vi "Temp_Calc.vi"(0 "aDATA":u8[](array[numeric])) -> (2 "Temp CH 1-4":dbl format="%#_3f", 3 "Temp CH 5-8":dbl, 4 "CPU Temp":dbl)   [LabVIEW 2010]
uses:
  <vilib>/Analysis/NI_AALPro.lvlib
panel:
  out "RT (Ohms) 2":dbl
  out "RT (Ohms)":dbl
  out "RT":dbl[](array[numeric]) format="%0.2f"
  out "Temp":dbl[](array[numeric]) format="%0.2f"
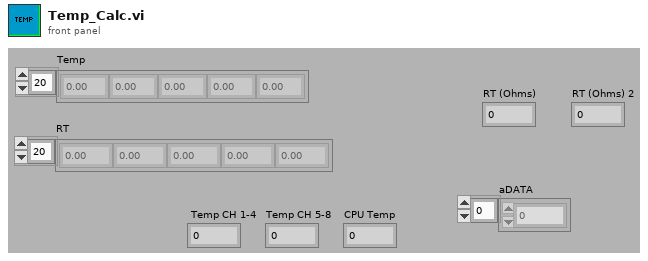
[diagram p1: front panel]
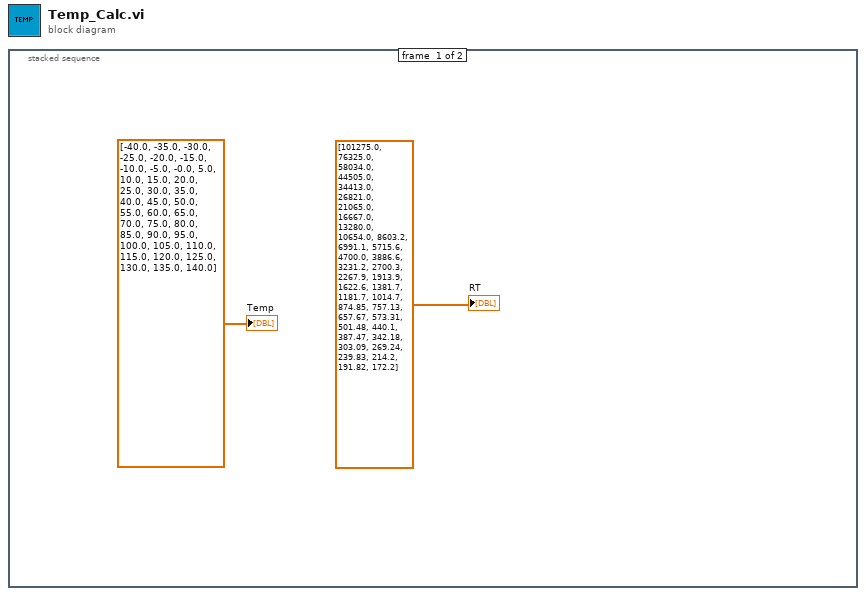
[diagram p0: block diagram]
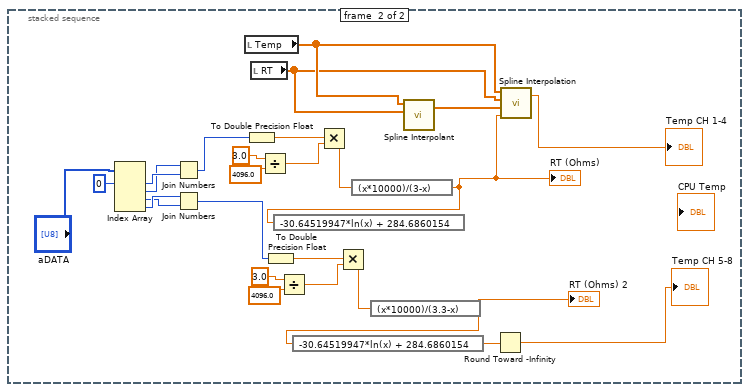
[diagram p2: hidden frame]
diagram:
  n1 = stacked-sequence {
    frame #0 {
      "Temp" <- dbl[] [-40.0, -35.0, -30.0, -25.0, -20.0, -15.0, -10.0, -5.0, -0.0, 5.0, 10.0, 15.0, 20.0, 25.0, 30.0, 35.0, 40.0, 45.0, 50.0, 55.0, 60.0, 65.0, 70.0, 75.0, 80.0, 85.0, 90.0, 95.0, 100.0, 105.0, 110.0, 115.0, 120.0, 125.0, 130.0, 135.0, 140.0] ("Temp")
      "RT" <- dbl[] [101275.0, 76325.0, 58034.0, 44505.0, 34413.0, 26821.0, 21065.0, 16667.0, 13280.0, 10654.0, 8603.2, 6991.1, 5715.6, 4700.0, 3886.6, 3231.2, 2700.3, 2267.9, 1913.9, 1622.6, 1381.7, 1181.7, 1014.7, 874.85, 757.13, 657.67, 573.31, 501.48, 440.1, 387.47, 342.18, 303.09, 269.24, 239.83, 214.2, 191.82, 172.2] ("RT")
    }
    frame #1 {
      n2 = Index Array(array="aDATA", index #1=0 ("index")) -> (element #1=w7:u8, element #2=w6:u8, element #3=w4:u8, element #4=w5:u8)  [unwired: 3 in]
      n3 = Join Numbers(hi=w6, lo=w7) -> ((hi.lo)=w12:u16)
      n4 = Join Numbers(hi=w5, lo=w4) -> ((hi.lo)=w20:u16)
      n5 = local read "Temp"() -> (w28:dbl[])
      n6 = To Double Precision Float(number=w12) -> (double precision float=w24:dbl)
      n7 = local read "RT"() -> (w27:dbl[])
      n8 = Divide(x=3.0, y=4096.0) -> (x/y=w9:dbl)
      n9 = To Double Precision Float(number=w20) -> (double precision float=w18:dbl)
      n10 = Divide(x=3.0, y=4096.0) -> (x/y=w15:dbl)
      n11 = Multiply(x=w24, y=w9) -> (x*y=w13:dbl)
      n12 = Multiply(x=w18, y=w15) -> (x*y=w19:dbl)
      n13 = expression code="(x*10000)/(3-x)"(w13) -> (w25:dbl)
      "RT (Ohms)" <- w25
      n14 = expression code="-30.64519947*ln(x) + 284.6860154"(w25) -> ()  [unwired: 1 out]
      n15 = expression code="(x*10000)/(3.3-x)"(w19) -> (w21:dbl)
      "RT (Ohms) 2" <- w21
      n16 = expression code="-30.64519947*ln(x) + 284.6860154"(w21) -> (w14:dbl)
      n17 = call <vilib>:"Spline Interpolant.vi"("X"=w27, "Y"=w28) -> ("Interpolant"=w23:dbl[])  [unwired: 2 in, 1 out]
      n18 = Round Toward -Infinity(1:w14) -> (0:→"Temp CH 5-8":dbl)
      n19 = call <vilib>:"Spline Interpolation.vi"("x value"=w25, "Interpolant"=w23, "X"=w27, "Y"=w28) -> ("interpolation value"=→"Temp CH 1-4":dbl)  [unwired: 1 out]
    }
  }
